vi "MOCKBEAR_Resample.vi"(8 "error in (no error)":errorcluster, 10 "FEA_Model in":refnum<class "FEA_Model.lvclass">, 11 "MOCKBEAR in":refnum<class "MOCKBEAR.lvclass">) -> (0 "error out":errorcluster, 3 "MOCKBEAR out":refnum<class "MOCKBEAR.lvclass">)   [LabVIEW 2021, in "MOCKBEAR.lvclass"]
uses:
  MOCKBEAR.lvclass
  FEA_Model/FEA_Model.lvclass
panel:
  out "Array":dbl[](array[numeric])
  in  "FFT Window":i32
  in  "New sample rate":dbl
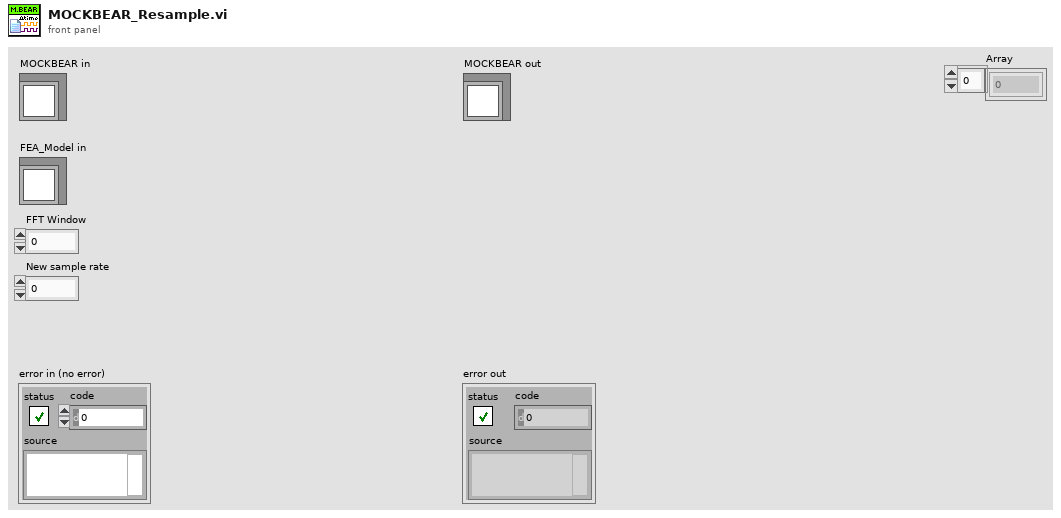
[diagram p1: front panel]
types:
  T1 = enum16{"Scalar Particle to Meter", "Scalar Node to Meter", "Scalar Meter to Particle", "Scalar Meter to Node", "Array Particle to Meter", "Array Node to Meter", "Array Meter to Particle", "Array Meter to Node"}
  T2 = enum16{"Recorded", "Auto Resample", "Custom Resample"}
  T3 = cluster{"Modeling Parameters":cluster{"beam_length":dbl, "youngs_modulus":dbl, "torsion_spring":dbl, "beam_height":dbl, "beam_width":dbl, "beam_density":dbl, "number_of_FEA_nodes":i32, "accelerometer_mass":dbl, "M Matrix":dbl[][], "K Matrix":dbl[][], "nodes_of_interest":i32[], "all_nodes":i32[]}, "Simulation Parameters":cluster{"Eigensolver ":enum16{"LabVIEW Cholesky", "LabVIEW General", "LabVIEW Inverse", "LEMP"}, "Pin Estimate":i32, "Frequency Estimate":dbl, "Models Forcasted":i32, "Max frequency":dbl, "Min frequency":dbl, "Frequency delta per node":dbl, "Max frequency delta per second":dbl, "Max Roller Velocity":dbl, "Max Roller Position Percent":dbl, "Min Roller Position Percent":dbl, "Particle Frequencies":dbl[], "Particles":i32[], "Particles Positions":dbl[], "Frequency Target":dbl, "Position estimate":dbl}, "LEMP":cluster{"Eigenvalues":dbl[], "SquareT Eigenvectors":dbl[][], "1/deltaStiff":dbl}}
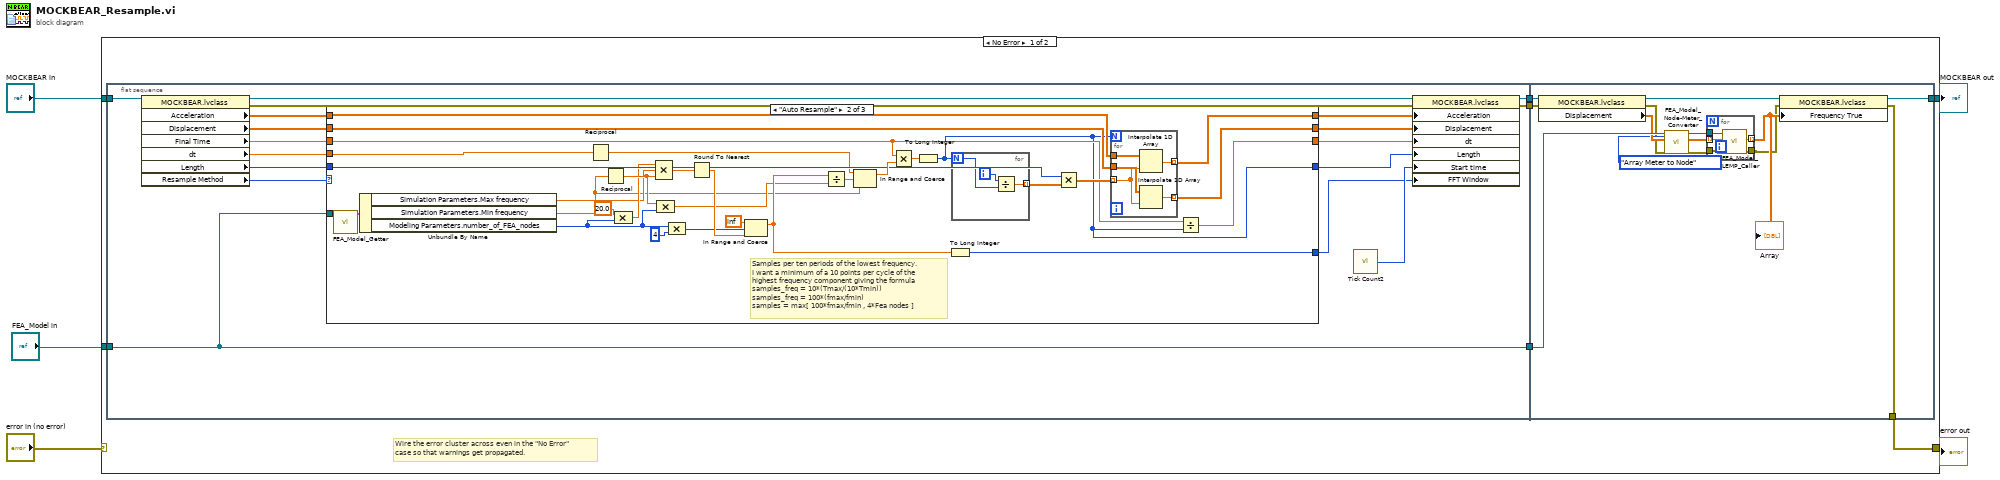
[diagram p0: block diagram]
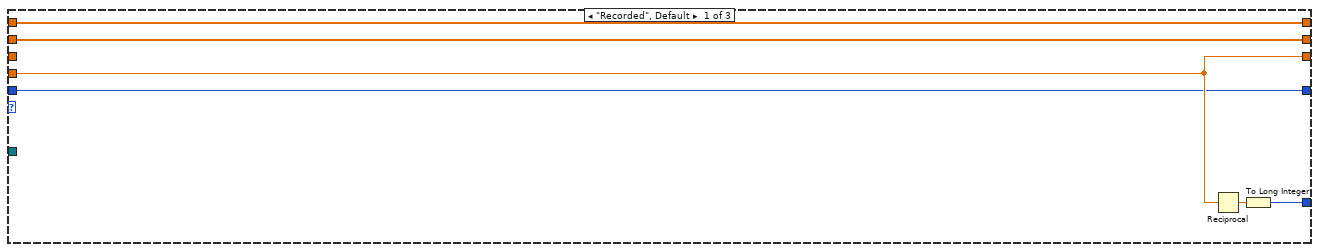
[diagram p2: hidden frame]
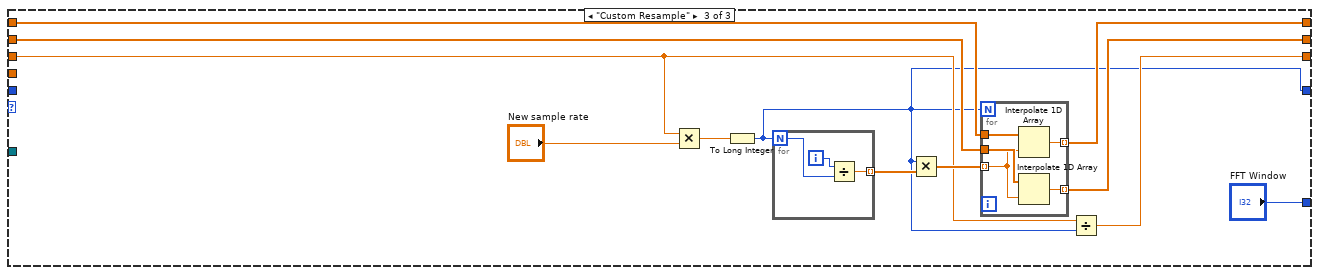
[diagram p3: hidden frame]
diagram:
  n1 = case shown="No Error" "error in (no error)" {
    selector: "error in (no error)" -> [_ w116]
    tunnel: [w6 w116] -> w4
    tunnel: [w11 w115] -> w2
    tunnel: "MOCKBEAR in" -> [w12 w115]
    tunnel: "FEA_Model in" -> [w10 _]
    frame No Error {
      # "Wire the error cluster across even in the \"No Error\"\ncase so that warnings get propagated."
      n2 = flat-sequence {
        tunnel: w12 -> [w17]
        tunnel: w10 -> [w13]
        tunnel: [w18] -> w9
        tunnel: [w14] -> w8
        tunnel: [w13] -> w7
        tunnel: [w101] -> w11
        tunnel: w9 -> [w109]
        tunnel: w8 -> [w108]
        tunnel: w7 -> [w107]
        tunnel: [w96] -> w6
        frame #0 {
          n3 = property class="MOCKBEAR.lvclass"(reference=w17) -> (reference out=w16:refnum<class "MOCKBEAR.lvclass">, error out=w15:errorcluster, "Acceleration"=w30:dbl[], "Displacement"=w29:dbl[], "Final Time"=w28:dbl, "dt"=w27:dbl, "Length"=w26:i32, "Resample Method"=w25:T2)  [unwired: 1 in]
          n4 = case shown="\"Auto Resample\"" w25 {
            tunnel: [w34 w64 "FFT Window"] -> w19
            tunnel: [w33 w63 w81] -> w22
            tunnel: [w35 w62 w82] -> w23
            tunnel: [w36 w61 w83] -> w24
            tunnel: w30 -> [w36 w58 w85]
            tunnel: w29 -> [w35 w57 w84]
            tunnel: w26 -> [w32 w56 _]
            tunnel: w28 -> [_ w55 w80]
            tunnel: w27 -> [w33 w54 _]
            tunnel: [w32 w42 w77] -> w21
            tunnel: w13 -> [_ w41 _]
            frame "Recorded", Default {
              n5 = Reciprocal(x=w33) -> (1/x=w31:dbl)
              n6 = To Long Integer(number=w31) -> (32bit integer=w34:i32)
            }
            frame "Auto Resample" {
              # "Samples per ten periods of the lowest frequency. \nI want a minimum of a 10 points per cycle of the \nhighest frequency component giving the formula\nsamples_freq = 10*(Tmax/(10*Tmin)) \nsamples_freq = 100*(fmax/fmin)\nsamples = max[ 100*fmax/fmin , 4*Fea nodes ]"
              n7 = call-dynamic "FEA_Model_Getter.vi"("FEA_Model in"=w41) -> ("FEA Model"=w40:T3)  [unwired: 9 in, 1 out]
              n8 = Unbundle By Name(w40) -> ("Simulation Parameters.Max frequency"=w39:dbl, "Simulation Parameters.Min frequency"=w38:dbl, "Modeling Parameters.number_of_FEA_nodes"=w37:i32)
              n9 = Reciprocal(x=w54) -> (1/x=w43:dbl)
              n10 = Reciprocal(x=w38) -> (1/x=w50:dbl)
              n11 = Compound Arithmetic op=MULTIPLY(20.0 ("value"), w37) -> (w46:dbl)
              n12 = Compound Arithmetic op=MULTIPLY(w46, w39, w50) -> (w53:dbl)
              n13 = Compound Arithmetic op=MULTIPLY(w50, w37) -> (w44:dbl)
              n14 = Compound Arithmetic op=MULTIPLY(w37, 4 ("Modeling Parameters.number_of_FEA_nodes")) -> (w51:i32)
              n15 = Round To Nearest(number=w53) -> (nearest integer value=w52:dbl)
              n16 = In Range and Coerce(upper limit=inf, x=w51, lower limit=w52) -> (coerced(x)=w60:dbl)  [unwired: 1 out]
              n17 = Divide(x=w60, y=w44) -> (x/y=w45:dbl)
              n18 = In Range and Coerce(upper limit=w43, x=w45, lower limit=w38) -> (coerced(x)=w59:dbl)  [unwired: 1 out]
              n19 = Multiply(x=w55, y=w59) -> (x*y=w65:dbl)
              n20 = To Long Integer(number=w65) -> (32bit integer=w42:i32)
              n21 = To Long Integer(number=w60) -> (32bit integer=w64:i32)
              n22 = for {
                N: w42 -> [w69]
                tunnel: [w68] -> w67 mode=indexing
                i -> [w70]
                n23 = Divide(x=w70, y=w69) -> (x/y=w68:dbl)
              }
              n24 = Multiply(x=w56, y=w67) -> (x*y=w66:dbl[])
              n25 = for {
                N: w42 -> [_]
                tunnel: w58 -> [w75]
                tunnel: w57 -> [w74]
                tunnel: w66 -> [w73] mode=indexing
                tunnel: [w72] -> w61 mode=indexing
                tunnel: [w71] -> w62 mode=indexing
                n26 = Interpolate 1D Array(1:w73, 2:w75) -> (0:w72:dbl)
                n27 = Interpolate 1D Array(1:w73, 2:w74) -> (0:w71:dbl)
              }
              n28 = Divide(x=w55, y=w42) -> (x/y=w63:dbl)
            }
            frame "Custom Resample" {
              n29 = Multiply(x=w80, y="New sample rate") -> (x*y=w78:dbl)
              n30 = To Long Integer(number=w78) -> (32bit integer=w77:i32)
              n31 = for {
                N: w77 -> [w89]
                tunnel: [w88] -> w87 mode=indexing
                i -> [w90]
                n32 = Divide(x=w90, y=w89) -> (x/y=w88:dbl)
              }
              n33 = Multiply(x=w77, y=w87) -> (x*y=w86:dbl[])
              n34 = for {
                N: w77 -> [_]
                tunnel: w85 -> [w95]
                tunnel: w84 -> [w94]
                tunnel: w86 -> [w93] mode=indexing
                tunnel: [w92] -> w83 mode=indexing
                tunnel: [w91] -> w82 mode=indexing
                n35 = Interpolate 1D Array(1:w93, 2:w95) -> (0:w92:dbl)
                n36 = Interpolate 1D Array(1:w93, 2:w94) -> (0:w91:dbl)
              }
              n37 = Divide(x=w80, y=w77) -> (x/y=w81:dbl)
            }
          }
          n38 = call "Tick Count2"() -> ("Tick Count(uSec)"=w20:u32)
          n39 = property class="MOCKBEAR.lvclass"(reference=w16, error in=w15, "Acceleration"=w24, "Displacement"=w23, "dt"=w22, "Length"=w21, "Start time"=w20, "FFT Window"=w19) -> (reference out=w18:refnum<class "MOCKBEAR.lvclass">, error out=w14:errorcluster)
        }
        frame #1 {
          n40 = property class="MOCKBEAR.lvclass"(reference=w109, error in=w108) -> (reference out=w102:refnum<class "MOCKBEAR.lvclass">, error out=w100:errorcluster, "Displacement"=w106:dbl[])
          n41 = call "FEA_Model_Node-Meter_Converter.vi"("Conversion Mode"=T1."Array Meter to Node", "error in (no error)"=w100, "Array in"=w106, "FEA_Model in"=w107) -> ("error out"=w99:errorcluster, "Array out"=w104:dbl[], "FEA_Model out"=w103:refnum<class "FEA_Model.lvclass">)  [unwired: 4 in, 1 out]
          n42 = for {
            tunnel: w104 -> [w114] mode=indexing
            tunnel: w103 -> [w113]
            tunnel: w99 -> [w112]
            tunnel: [w111] -> w98 mode=indexing
            tunnel: [w110] -> w97
            n43 = call-dynamic "FEA_Model_LEMP_Caller.vi"("error in (no error)"=w112, "Node of interest"=w114, "FEA_Model in"=w113) -> ("error out"=w110:errorcluster, "Frequency"=w111:dbl)  [unwired: 6 in, 1 out]
          }
          "Array" <- w98
          n44 = property class="MOCKBEAR.lvclass"(reference=w102, error in=w97, "Frequency True"=w98) -> (reference out=w101:refnum<class "MOCKBEAR.lvclass">, error out=w96:errorcluster)
        }
      }
    }
    frame Error {
    }
  }
  "error out" <- w4
  "MOCKBEAR out" <- w2
